vi "Init Tx - Dynamic Header.vi"(8 "error in (no error)":errorcluster, 11 "Tx Loop Data":T1) -> (0 "error out":errorcluster, 3 "Tx Loop Data out":T1)   [LabVIEW 2019, in "UDP-Custom-Device Engine.lvlib"]
uses:
  UDP-Custom-Device Engine.lvlib
  Types/Engine - Tx Loop Data.ctl
  <vilib>/NI VeriStand/VeriStand Data/Byte Buffer/Byte Buffer.lvclass
  Types/Engine - General Resources.ctl
  <vilib>/NI VeriStand/VeriStand Data/Typedefs/Typedefs.Data Types.ctl
  Shared/Types/Shared - Duplex Settings.ctl
  Shared/Types/Shared - Header Details.ctl
  Types/Engine - Data Conversion Config.ctl
  <vilib>/NI VeriStand/VeriStand Data/Byte Buffer/Byte Buffer.Mapping.ctl
  Types/Engine - Tx Runtime Resources.ctl
  Shared/Types/Shared - Transmit Flag Options.ctl
  Types/Engine - Execution Config.ctl
  Shared/Types/Shared - Thread Management.ctl
  Types/Engine - Tx Echo Resources.ctl
  Shared/Types/Shared - Transmit Echo Options.ctl
  Types/Engine - Tx Channel Refs.ctl
  <vilib>/NI/NIVS Inline Async API/_Data Access Engine/Data Access Engine/Types/Read.DVR.ctl
  <vilib>/NI/NIVS Inline Async API/_Data Access Engine/Access Type Classes/Read/Read.lvclass
  <vilib>/NI/NIVS Inline Async API/_Data Access Engine/Data Access Engine/Types/Write.DVR.ctl
  <vilib>/NI/NIVS Inline Async API/_Data Access Engine/Access Type Classes/Write/Write.lvclass
  Types/Engine - Debug Resources.ctl
  <vilib>/NI VeriStand/VeriStand Data/VeriStand Data.lvlib
  <vilib>/NI/NIVS Inline Async API/_Data Access Engine/Data Access Engine/Data Access Engine.lvclass
  Shared/UDP-Custom-Device Shared.lvlib
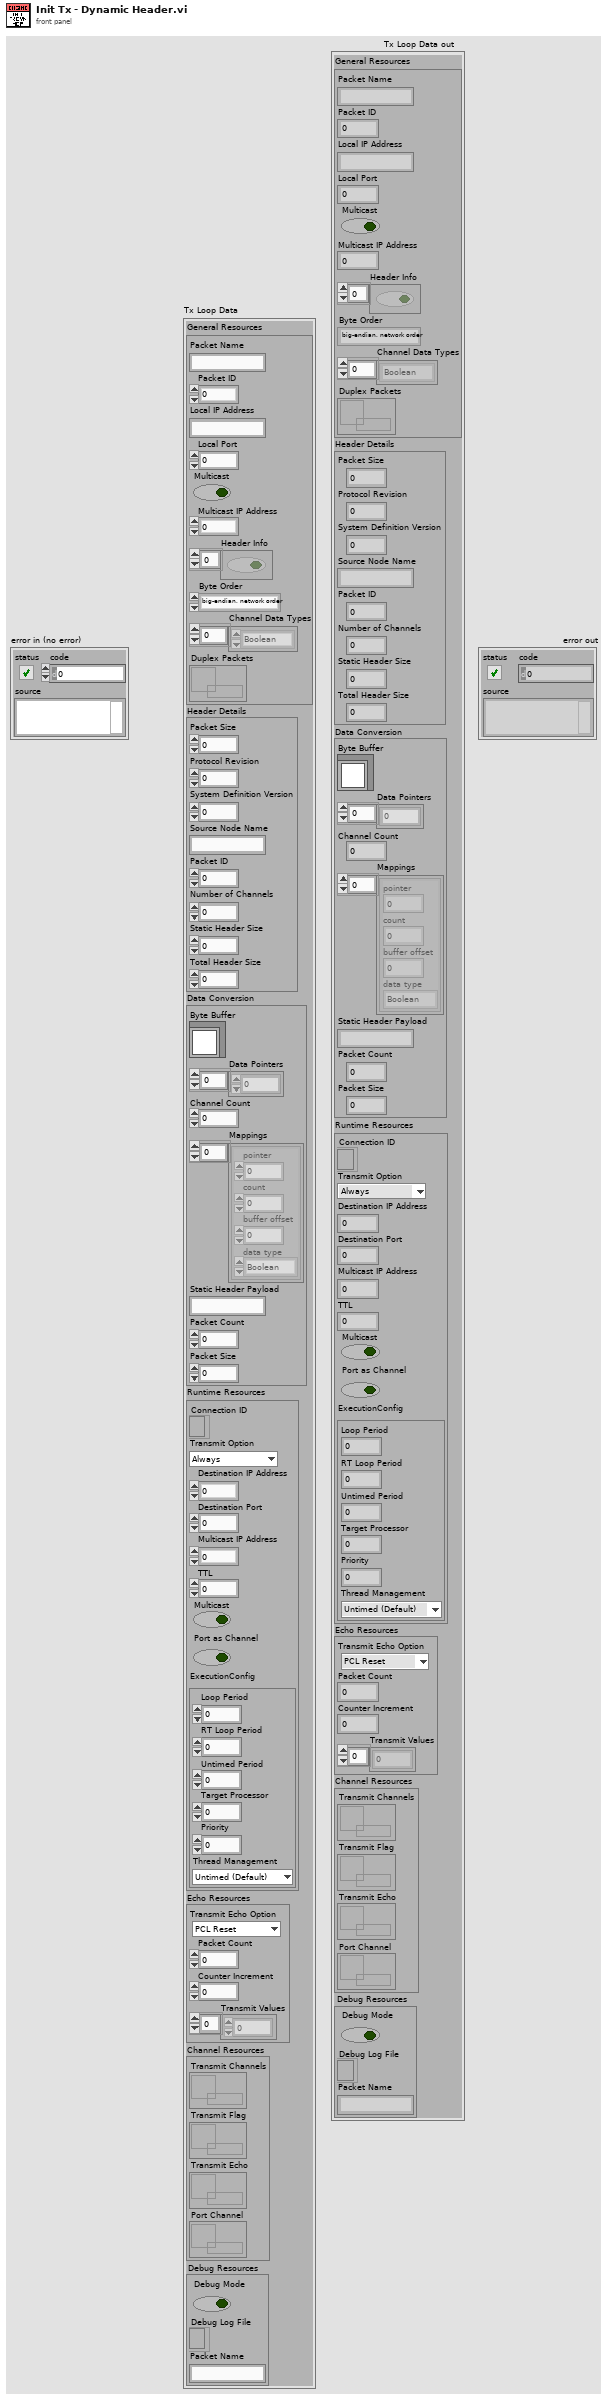
[diagram p1: front panel]
types:
  T1 = typedef "UDP-Custom-Device Engine.lvlib/Engine - Tx Loop Data.ctl" = cluster{"General Resources":T2, "Header Details":T4, "Data Conversion":T5, "Runtime Resources":T7, "Echo Resources":T11, "Channel Resources":T13, "Debug Resources":T16}
  T2 = typedef "UDP-Custom-Device Engine.lvlib/Engine - General Resources.ctl" = cluster{"Packet Name":string, "Packet ID":i32, "Local IP Address":string, "Local Port":i32, "Multicast":bool, "Multicast IP Address":u32, "Header Info":bool[], "Byte Order":enum16{"big-endian, network order", "native, host order", "little-endian"}, "Channel Data Types":T3[], "Duplex Packets":refnum<data-value>}
  T3 = typedef "VeriStand Data.lvlib/Typedefs.Data Types.ctl" = enum16{"Boolean", "Single", "Double", "I8", "I16", "I32", "I64", "U8", "U16", "U32", "U64"}
  T4 = typedef "UDP-Custom-Device Shared.lvlib/Shared - Header Details.ctl" = cluster{"Packet Size":u16, "Protocol Revision":u8, "System Definition Version":u64, "Source Node Name":string, "Packet ID":u32, "Number of Channels":u32, "Static Header Size":u16, "Total Header Size":u16}
  T5 = typedef "UDP-Custom-Device Engine.lvlib/Engine - Data Conversion Config.ctl" = cluster{"Byte Buffer":refnum<class "Byte Buffer.lvclass">, "Data Pointers":u64[], "Channel Count":i32, "Mappings":T6[], "Static Header Payload":string, "Packet Count":dbl, "Packet Size":i32}
  T6 = typedef "VeriStand Data.lvlib/Byte Buffer.lvclass/Byte Buffer.Mapping.ctl" = cluster{"pointer":u64, "count":i64, "buffer offset":u64, "data type":T3}
  T7 = typedef "UDP-Custom-Device Engine.lvlib/Engine - Tx Runtime Resources.ctl" = cluster{"Connection ID":refnum<k16>, "Transmit Option":T8, "Destination IP Address":u32, "Destination Port":u16, "Multicast IP Address":u32, "TTL":u16, "Multicast":bool, "Port as Channel":bool, "ExecutionConfig":T9}
  T8 = typedef "UDP-Custom-Device Shared.lvlib/Shared - Transmit Flag Options.ctl" = enum16{"Always", "One-Shot", "Toggle"}
  T9 = typedef "UDP-Custom-Device Engine.lvlib/Engine - Execution Config.ctl" = cluster{"Loop Period":i64, "RT Loop Period":i64, "Untimed Period":u32, "Target Processor":i32, "Priority":i32, "Thread Management":T10}
  T10 = typedef "UDP-Custom-Device Shared.lvlib/Shared - Thread Management.ctl" = enum16{"Untimed (Default)", "Timed (High Priority)"}
  T11 = typedef "UDP-Custom-Device Engine.lvlib/Engine - Tx Echo Resources.ctl" = cluster{"Transmit Echo Option":T12, "Packet Count":dbl, "Counter Increment":dbl, "Transmit Values":dbl[]}
  T12 = typedef "UDP-Custom-Device Shared.lvlib/Shared - Transmit Echo Options.ctl" = enum16{"PCL Reset", "Counter", "Mirror"}
  T13 = typedef "UDP-Custom-Device Engine.lvlib/Engine - Tx Channel Refs.ctl" = cluster{"Transmit Channels":T14, "Transmit Flag":T14, "Transmit Echo":T15, "Port Channel":T14}
  T14 = typedef "Data Access Engine.lvlib/Data Access Engine.lvclass/Read.DVR.ctl" = refnum<data-value>
  T15 = typedef "Data Access Engine.lvlib/Data Access Engine.lvclass/Write.DVR.ctl" = refnum<data-value>
  T16 = typedef "UDP-Custom-Device Engine.lvlib/Engine - Debug Resources.ctl" = cluster{"Debug Mode":bool, "Debug Log File":refnum<file>, "Packet Name":string}
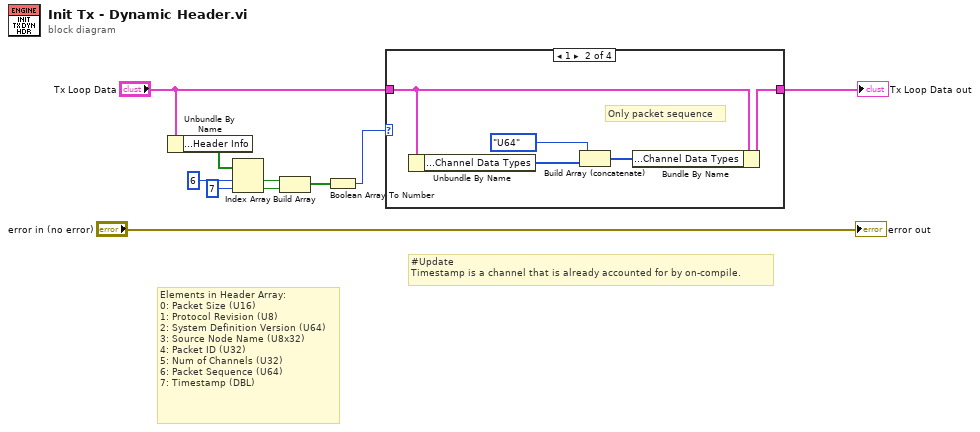
[diagram p0: block diagram]
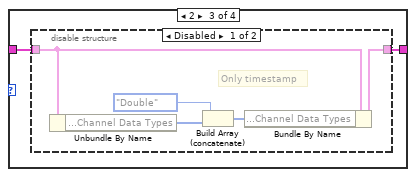
[diagram p3: hidden frame]
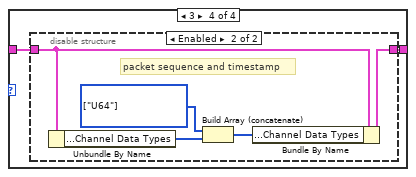
[diagram p5: hidden frame]
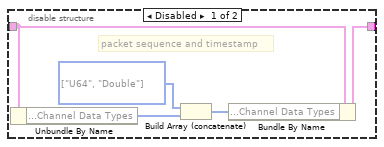
[diagram p6: hidden frame]
diagram:
  # "#Update\nTimestamp is a channel that is already accounted for by on-compile."
  # "Elements in Header Array:\n0: Packet Size (U16)\n1: Protocol Revision (U8)\n2: System Definition Version (U64)\n3: Source Node Name (U8x32)\n4: Packet ID (U32)\n5: Num of Channels (U32)\n6: Packet Sequence (U64)\n7: Timestamp (DBL)"
  n1 = Unbundle By Name("Tx Loop Data") -> ("General Resources.Header Info"=w7:bool[])
  n2 = Index Array(array=w7, index #1=6 ("index"), index #2=7 ("index")) -> (element #1=w4:bool, element #2=w3:bool)
  n3 = Build Array(w4, w3) -> (w2:bool[])
  n4 = Boolean Array To Number(Boolean array=w2) -> (number=w1:u32)
  n5 = case shown="1" w1 {
    tunnel: [w11 w13 w17 w25] -> w10
    tunnel: "Tx Loop Data" -> [w11 w14 w18 w26]
    frame 0, Default {
      # "No packet sequence or timestamp"
    }
    frame 1 {
      # "Only packet sequence"
      n6 = Unbundle By Name(w14) -> ("General Resources.Channel Data Types"=w16:T3[])
      n7 = Build Array (concatenate)(Typedefs.Data_Types."U64" ("data type"), w16) -> (w12:T3[])
      n8 = Bundle By Name(cluster=w14, "General Resources.Channel Data Types"=w12) -> (w13:T1)
    }
    frame 2 {
      n9 = disable-structure shown="Disabled" {
        disable-tunnel: w18 -> [w21 w24]
        disable-tunnel: [w20 w24] -> w17
        frame Disabled {
          # "Only timestamp"
          n10 = Unbundle By Name(w21) -> ("General Resources.Channel Data Types"=w23:T3[])
          n11 = Build Array (concatenate)(Typedefs.Data_Types."Double" ("data type"), w23) -> (w19:T3[])
          n12 = Bundle By Name(cluster=w21, "General Resources.Channel Data Types"=w19) -> (w20:T1)
        }
        frame Enabled {
        }
      }
    }
    frame 3 {
      n13 = disable-structure shown="Enabled" {
        disable-tunnel: w26 -> [w30 w35]
        disable-tunnel: [w29 w34] -> w25
        frame Disabled {
          w27 = T3[] [enum."U64", enum."Double"] items=["Boolean", "Single", "Double", "I8", "I16", "I32", "I64", "U8", "U16", "U32", "U64"] ("Array")
          # "packet sequence and timestamp"
          n14 = Unbundle By Name(w30) -> ("General Resources.Channel Data Types"=w31:T3[])
          n15 = Build Array (concatenate)(w27, w31) -> (w28:T3[])
          n16 = Bundle By Name(cluster=w30, "General Resources.Channel Data Types"=w28) -> (w29:T1)
        }
        frame Enabled {
          w32 = T3[] [enum."U64"] items=["Boolean", "Single", "Double", "I8", "I16", "I32", "I64", "U8", "U16", "U32", "U64"] ("Array")
          # "packet sequence and timestamp"
          n17 = Unbundle By Name(w35) -> ("General Resources.Channel Data Types"=w36:T3[])
          n18 = Build Array (concatenate)(w32, w36) -> (w33:T3[])
          n19 = Bundle By Name(cluster=w35, "General Resources.Channel Data Types"=w33) -> (w34:T1)
        }
      }
    }
  }
  "Tx Loop Data out" <- w10
  "error out" <- "error in (no error)"
